vi "개별읽기요구(subVI).vi"(1 "직접변수":string[](array[string])) -> (0 "개별읽기":string)   [LabVIEW 2014]
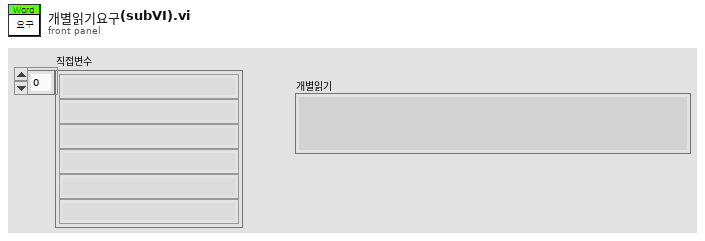
[diagram p1: front panel]
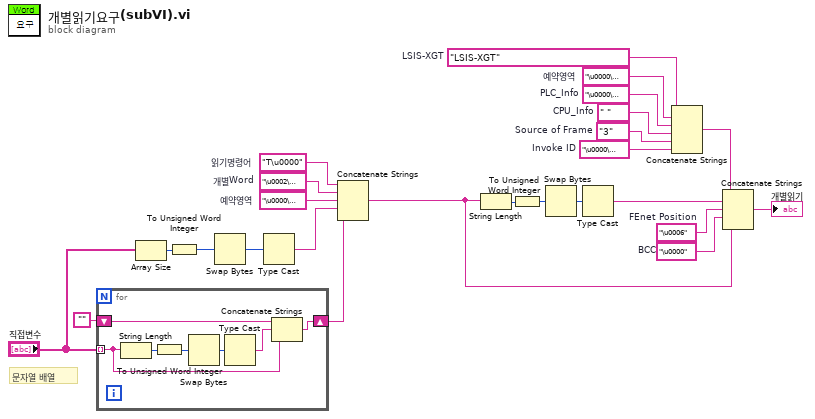
[diagram p0: block diagram]
diagram:
  w9 = "\u0000"  # BCC
  w10 = "\u0006"  # FEnet Position
  w13 = "\u0000\u0000"  # Invoke ID
  w14 = "3"  # Source of Frame
  w15 = " "  # CPU_Info
  w16 = "\u0000\u0000"  # PLC_Info
  w17 = "\u0000\u0000"  # 예약영역
  w18 = "LSIS-XGT"  # LSIS-XGT
  w23 = "\u0000\u0000"  # 예약영역
  w24 = "\u0002\u0000"  # 개별Word
  w25 = "T\u0000"  # 읽기명령어
  # "문자열 배열"
  n1 = for {
    shift-right: [w32] -> w19
    shift-left: "" -> [w29]
    tunnel: "직접변수" -> [w30] mode=indexing
    n2 = String Length(string=w30) -> (length=w31:i32)
    n3 = To Unsigned Word Integer(number=w31) -> (unsigned 16bit integer=w27:u16)
    n4 = Swap Bytes(anything=w27) -> (byte swapped=w28:u16)
    n5 = Type Cast(x=w28) -> (*(type *) &x=w26:string)  [unwired: 1 in]
    n6 = Concatenate Strings(w29, w26, w30) -> (w32:string)
  }
  n7 = Array Size(array="직접변수") -> (size(s)=w22:i32)
  n8 = To Unsigned Word Integer(number=w22) -> (unsigned 16bit integer=w2:u16)
  n9 = Swap Bytes(anything=w2) -> (byte swapped=w3:u16)
  n10 = Type Cast(x=w3) -> (*(type *) &x=w1:string)  [unwired: 1 in]
  n11 = Concatenate Strings(w25, w24, w23, w1, w19) -> (w11:string)
  n12 = String Length(string=w11) -> (length=w7:i32)
  n13 = To Unsigned Word Integer(number=w7) -> (unsigned 16bit integer=w6:u16)
  n14 = Swap Bytes(anything=w6) -> (byte swapped=w5:u16)
  n15 = Type Cast(x=w5) -> (*(type *) &x=w4:string)  [unwired: 1 in]
  n16 = Concatenate Strings(w18, w17, w16, w15, w14, w13) -> (w12:string)
  n17 = Concatenate Strings(w12, w4, w10, w9, w11) -> (→"개별읽기":string)
